vi "Dashboard Main.vi"() -> ()   [LabVIEW 2019]
uses:
  <vilib>/Rock Robotics/Network Tables/NT Read Numeric Array.vi
  <vilib>/Rock Robotics/Network Tables/NT Read String.vi
  <vilib>/Rock Robotics/Network Tables/NT Read Number.vi
  <vilib>/Rock Robotics/Network Tables/NT Read Boolean.vi
  <vilib>/Rock Robotics/Network Tables/NT Write Number.vi
panel:
  out "Camera Perf":string
  in  "Camera Settings":T1={"Frame Rate"=30, "Compression"=30, "Size"=1, "DB Camera Config"=FALSE} {"Frame Rate" scale=1.0..30.0; "Compression" scale=100.0..-1.0; "Size" items=["640x480", "320x240", "160x120"]}
  in  "TCP":refnum<k5>
  out "Robot IP":string
  in  "Dashboard Tab":T2(tab)
  in  "Select Auto":string(combo)="Select Autonomous ..."
  out "NT Connection":bool
  out "MotorChart R":cluster{"Numeric":dbl, "Numeric":dbl}(graph)
  out "MotorChart L":cluster{"Numeric":dbl, "Numeric":dbl}(graph)
  out "MotorSliders R":cluster{"MotorSlide1":dbl, "MotorSlide2":dbl} {"MotorSlide2" scale=-1.0..1.0 scale format="%#_2e"; "MotorSlide1" scale=-1.0..1.0 scale format="%#_2e"}
  out "MotorSliders L":cluster{"MotorSlide1":dbl, "MotorSlide2":dbl} {"MotorSlide2" scale=-1.0..1.0 scale format="%#_2e"; "MotorSlide1" scale=-1.0..1.0 scale format="%#_2e"}
  out "JS1 Z":dbl(slide) scale=-1.0..1.0 scale format="%#_2e"
  out "JS1 Graph":cluster{"X":dbl, "Y":dbl}[](graph)
  out "JS1 Buttons":T3
  out "JS2 Z":dbl(slide) scale=-1.0..1.0 scale format="%#_2e"
  out "JS2 Graph":cluster{"X":dbl, "Y":dbl}[](graph)
  out "JS2 Buttons":T3
  out "Mode":T4(ring)=enum."Auto Disabled"
  in  "Camera Name 2":string(combo)="No Camera Selection"
  out "Camera Image 2":T5(plugin-control)
  out "Target Spotted":bool
  out "Color Box":u32(colorbox)
  out "New Center Y":dbl
  out "New Center X":dbl
  out "y change":dbl
  out "Top Left Y":dbl
  out "Bottom Right Y":dbl
  out "Bottom Right X":dbl
  out "Top left X":dbl
  out "x change":dbl
  out "full angle":dbl
  in  "RectHeight":dbl
  in  "RectWidth":dbl
  in  "RectAngle":dbl
  in  "RectY":dbl
  in  "RectX":dbl
  out "Distance Formula 2":dbl
  out "Distance Formula 1":dbl
  out "Bottom Left Y":dbl
  out "Bottom Left X":dbl
  out "Top Right X":dbl
  out "Top Right Y":dbl
  out "New Full Angle":dbl
  out "2nd Y Change":dbl
  out "2nd X Change":dbl
  out "Final Center Y":dbl
  out "Final Center X":dbl
  out "Robot Angle":dbl
  out "Right Target":dbl
  out "Left Target":dbl
  out "Average Distance":dbl
  out "Right Distance":dbl
  out "Left Distance":dbl
  out "Right Speed":dbl
  out "Average Speed":dbl
  out "Left Speed":dbl
  out "Left":dbl[](graph)
  out "Right":dbl[](graph)
  out "Current Filter":T6 {"Value" scale=0.0..255.0; "Saturation" scale=0.0..255.0; "Hue" scale=0.0..255.0}
  in  "Update Filter":bool
  in  "New Filter":T6 {"Value" scale=0.0..255.0; "Saturation" scale=0.0..255.0; "Hue" scale=0.0..255.0}
  out "RectX":dbl
  out "RectY":dbl
  out "RectAngle":dbl
  out "RectWidth":dbl
  out "RectHeight":dbl
  out "left y":dbl
  out "right y":dbl
  out "right x":dbl
  out "left x":dbl
  in  "Update":bool
  in  "Kd":dbl format="%10.0f"
  in  "Ki":dbl format="%10.0f"
  in  "Kp":dbl format="%10.0f"
  in  "Kf":dbl format="%10.0f"
  out "Right Speed 2":dbl format="%10.0f"
  out "Left Speed 2":dbl format="%10.0f"
  out "Waveform Chart":dbl[](graph)
  in  "Right Dmd":dbl format="%10.0f"
  in  "Left Dmd":dbl format="%10.0f"
  out "Tree":string(tree)
  out "Camera Image":T5(plugin-control)
  out "Background":bool
  in  "Camera Name":string(combo)="No Camera Selection"
  # "HW"
  # "Joysticks"
  # "Drive Motors"
  # "Front"
  # "Right"
  # "Left"
  # "Back"
  # "Target Spotted"
  # "Color Sensor 90 Degree Color"
  # "Left"
  # "Right"
  # "Average"
  # "Speed"
  # "Target Speed"
  # "Distance"
  # "Robot Angle"
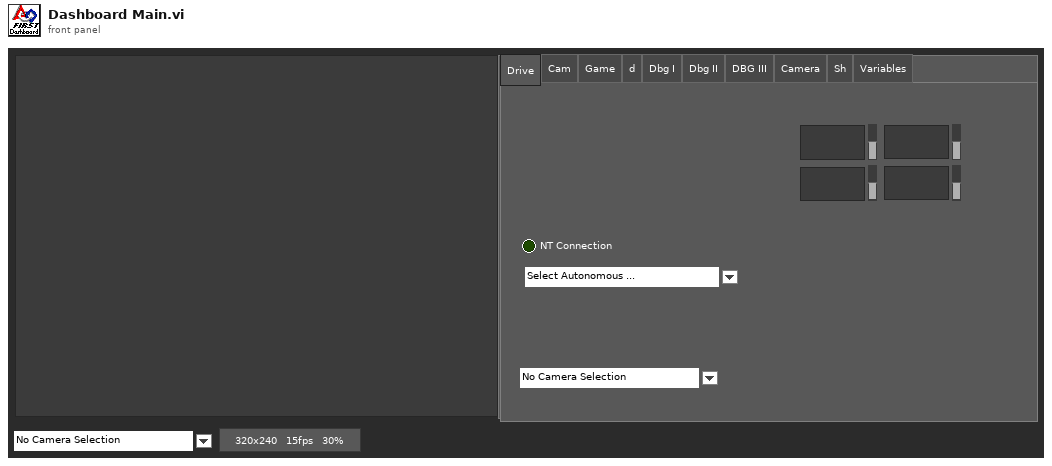
[diagram p1: front panel]
types:
  T1 = cluster{"Frame Rate":i32, "Compression":i32, "Size":u16, "DB Camera Config":bool}
  T2 = enum32{"Drive", "Cam", "Game", "d", "Dbg I", "Dbg II", "DBG III", "Camera", "Sh", "Variables"}
  T3 = cluster{bool, bool, bool, bool, bool, bool, bool, bool, bool, bool, bool, bool}
  T4 = enum8{"Tele-Op Disabled", "Tele-Op Enabled", "Auto Disabled", "Auto Enabled", "Test Disabled", "Test Enabled", "Disconnected", "No Code", "E-Stop"}
  T5 = typedef "IMAQ Image.ctl" = refnum<image>
  T6 = cluster{"Hue":cluster{dbl, dbl}, "Saturation":cluster{dbl, dbl}, "Value":cluster{dbl, dbl}}
  T7 = typedef "Image Type" = u32
  T8 = cluster{"Save Path":path, "Interval (s)":dbl, "Keep":i32}
  T9 = cluster{"Camera Image":refnum<vi>, "Dashboard Tab":refnum<vi>, "Background":refnum<vi>, "Tree":refnum<vi>, "Camera Settings":refnum<vi>, "Camera Name":refnum<vi>, "Camera Perf":refnum<vi>}
  T10 = cluster{"Shift":bool, "Ctrl":bool, "Alt":bool, "Cmd":bool, "Opt":bool}
  T11 = cluster{"Camera Name":string, "Camera File Name":string, "Saved DB Images Info":cluster{"Save Path":path, "Interval (s)":dbl, "Keep":i32}}
  T12 = cluster{"left x":dbl, "left y":dbl, "right x":dbl, "right y":dbl}
  T13 = cluster{cluster{dbl, dbl}, cluster{dbl, dbl}, cluster{dbl, dbl}}
  T14 = cluster{"left x":dbl, "right y":dbl, "right x":dbl, "left y":dbl}
  T15 = cluster{"Camera Name 2":string, string, "Saved DB Images Info":cluster{"Save Path":path, "Interval (s)":dbl, "Keep":i32}}
  T16 = cluster{"Error Strings":string, "Disable Counts":cluster{u16, u16}, "Rail Faults":cluster{u16, u16, u16}, "Robot IP":string, "DB Mode":u8, "Event Info":cluster{"Name":string, "Type":u8, "Number":u16, "Replay":u8}}
  T17 = cluster{"Storage":cluster{"Disk Free":u64, "RAM Block":u32, "RAM free":u32}, "CPU Utilization":cluster{"CPU % ISR":sgl, "CPU % Time Crit":sgl, "CPU % Timed Str":sgl, "CPU % High":sgl, "CPU % Above":sgl, "CPU % Normal":sgl, "CPU % Low":sgl}, "CAN":cluster{"% Bus Utilization":sgl, "Bus Off Cnt":u32, "TX_FIFO Full Cnt":u32, "Receive Error Cnt":u8, "Transmit Error Cnt":u8}, "HID":cluster{"HID Outputs":u32, "Rumble Low":u16, "Rumble High":u16}[]}
  T18 = cluster{"Status bits":cluster{"Test Mode":bool, "Autonomous":bool, "Enabled":bool, "Code Start":bool, "Brownout":bool, "Reserved 2":bool, "Reserved 3":bool, "E-Stop":bool}, "Code Trace":cluster{"Disabled":bool, "TeleOp":bool, "Auto":bool, "Test":bool}, "Controller Type":enum16{"unknown", "cRIO", "roboRio"}, "Code?":enum16{"unknown", "noCode", "code"}, "Battery V":dbl}
  T19 = cluster{"Control Bits":cluster{"TestMode":bool, "Autonomous":bool, "Enabled":bool, "FMS Present":bool, bool, bool, bool, "E-Stop":bool}, "Team Station ":u8, "Countdown":sgl, "Joystick Values":cluster{"Axes":dbl[], "Buttons":bool[], "POVs":i16[]}[]}
  T20 = cluster{"Axes":dbl[], "Buttons":bool[], "POVs":i16[]}[]
  T21 = cluster{"Axes":dbl[], "Buttons":bool[], "POVs":i16[]}
  T22 = cluster{"Buttons[0]":bool, "Buttons[1]":bool, "Buttons[2]":bool, "Buttons[3]":bool, "Buttons[4]":bool, "Buttons[5]":bool, "Buttons[6]":bool, "Buttons[7]":bool, "Buttons[8]":bool, "Buttons[9]":bool, "Buttons[10]":bool, "Buttons[11]":bool}
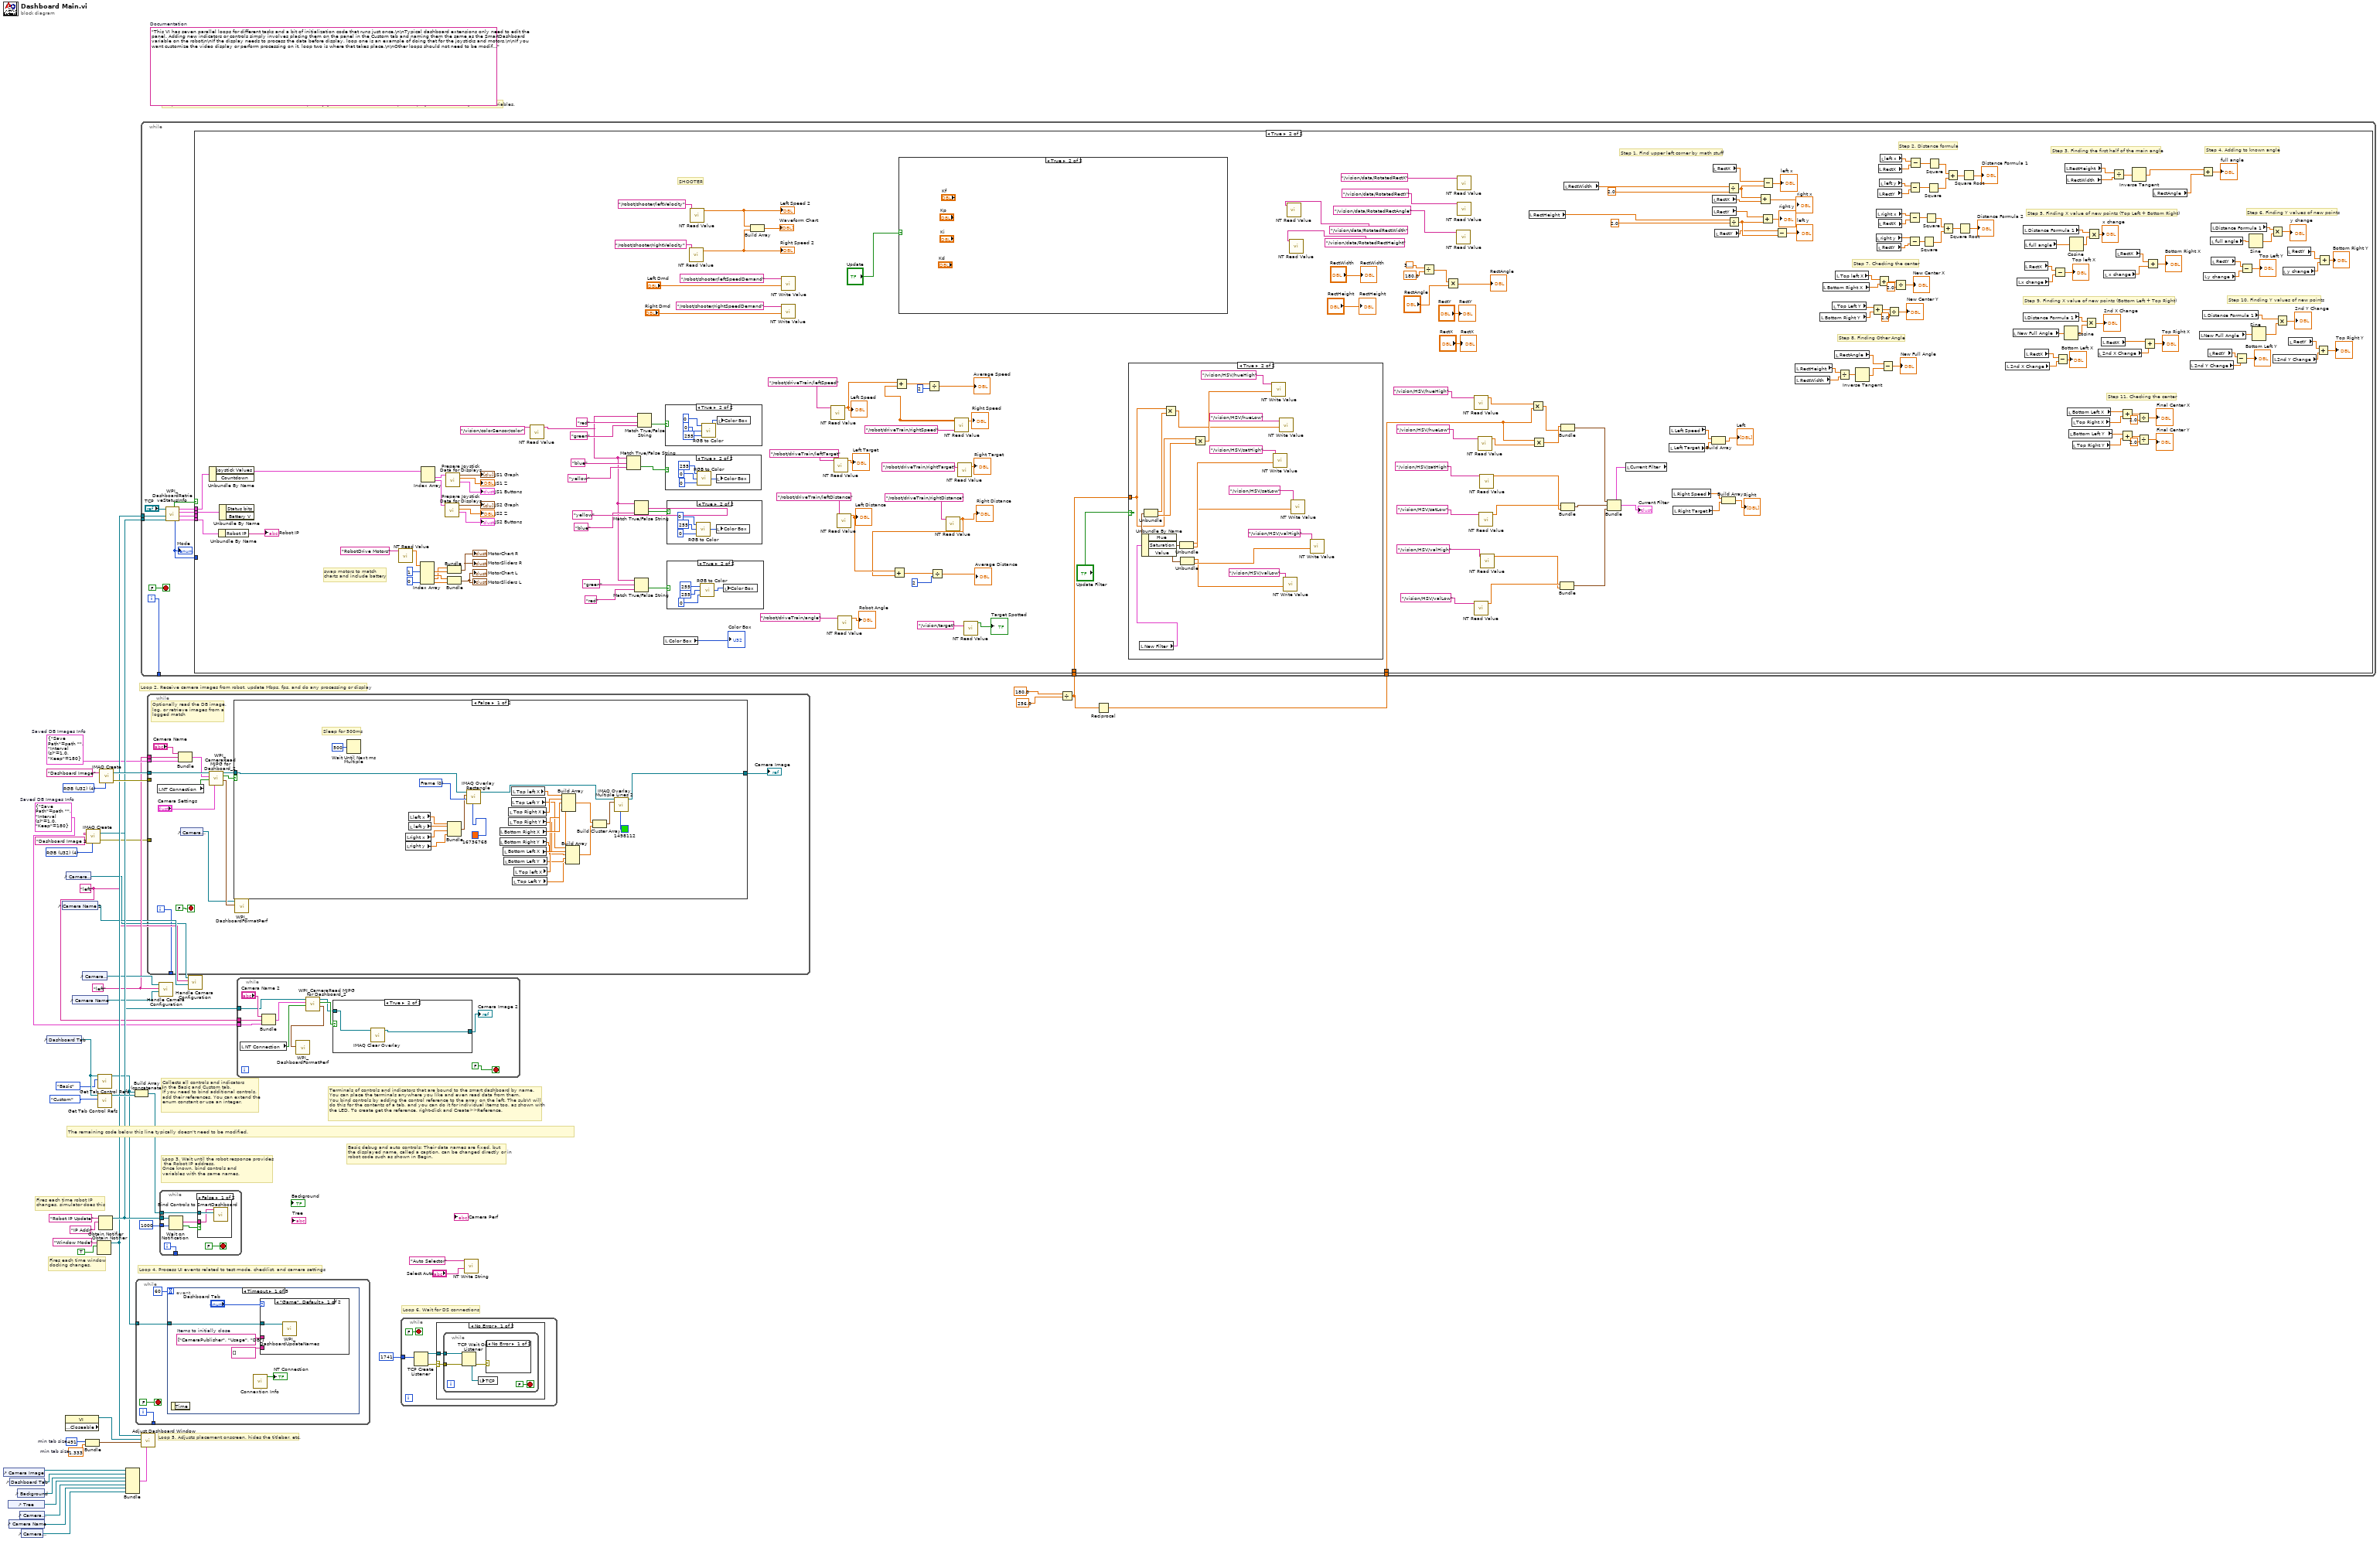
[diagram p0: block diagram]
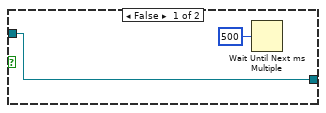
[diagram p2: hidden frame]
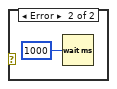
[diagram p3: hidden frame]
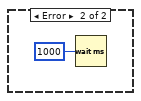
[diagram p4: hidden frame]
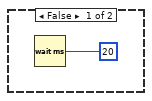
[diagram p5: hidden frame]
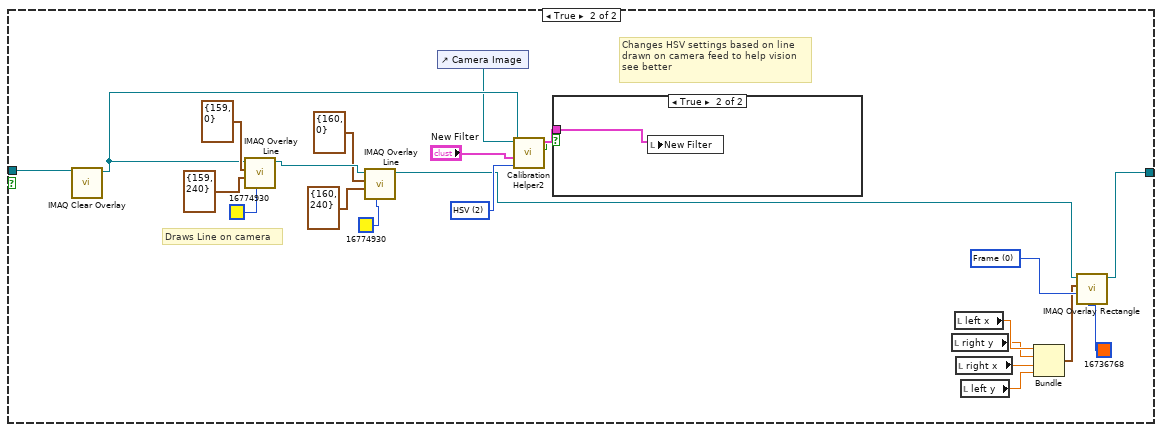
[diagram p13: hidden frame]
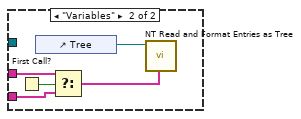
[diagram p15: hidden frame]
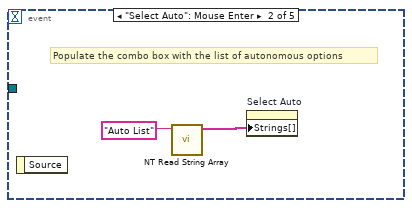
[diagram p16: hidden frame]
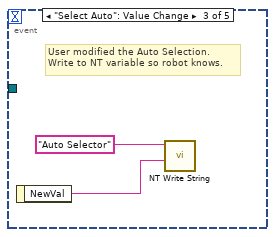
[diagram p17: hidden frame]
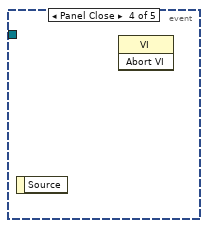
[diagram p18: hidden frame]
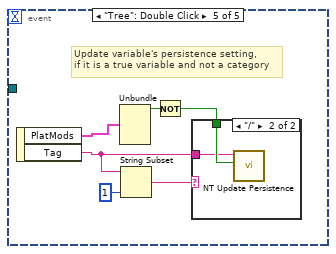
[diagram p19: hidden frame]
diagram:
  w5 = T7 4 items=["Grayscale (U8)", "Grayscale (I16)", "Grayscale (SGL)", "Complex (CSG)", "RGB (U32)", "HSL (U32)", "RGB (U64)"] ("Image Type")
  w2 = T8 {"Save Path"=path "", "Interval (s)"=1.0, "Keep"=180}  # Saved DB Images Info
  w3 = "left"
  w13 = "left" ("Camera File Name")
  w14 = T8 {"Save Path"=path "", "Interval (s)"=1.0, "Keep"=180}  # Saved DB Images Info
  w33 = 491  # min tab size
  w32 = 1.333  # min tab size
  (unwired) "This VI has seven parallel loops for different tasks and a bit of initialization code that runs just once.\n\nTypical dashboard extensions only need to edit the panel. Adding new indicators or controls simply involves placing them on the panel in the Custom tab and naming them the same as the SmartDashboard variable on the robot\n\nIf the display needs to process the data before display, loop one is an example of doing that for the joysticks and motors.\n\nIf you want customize the video display or perform processing on it, loop two is where that takes place.\n\nOther loops should not need to be modified. They are pretty standard, and document the task they perform."  # Documentation
  w48 = T7 4 items=["Grayscale (U8)", "Grayscale (I16)", "Grayscale (SGL)", "Complex (CSG)", "RGB (U32)", "HSL (U32)", "RGB (U64)"] ("Image Type")
  # "Terminals of controls and indicators that are bound to the smart dashboard by name.\nYou can place the terminals anywhere you like and even read data from them.\nYou bind controls by adding the control reference to the array on the left. The subVI will\ndo this for the contents of a tab, and you can do it for individual items too, as shown with\nthe LED. To create get the reference, right-click and Create>>Reference."
  # "Loop 6. Wait for DS connections"
  # "Basic debug and auto controls: Their data names are fixed, but\nthe displayed name, called a caption, can be changed directly or in\nrobot code such as shown in Begin."
  # "Fires each time robot IP\nchanges, simulator does this"
  # "Fires each time window\ndocking changes."
  # "Collects all controls and indicators\nin the Basic and Custom tab.\nIf you need to bind additional controls,\nadd their references. You can extend the\nenum constant or use an integer."
  # "The remaining code below this line typically doesn't need to be modified."
  # "Loop 4. Process UI events related to test mode, checklist, and camera settings"
  # "Loop 3. Wait until the robot response provides\n the Robot IP address.\nOnce known, bind controls and\nvariables with the same names."
  # "Loop 5. Adjusts placement onscreen, hides the titlebar, etc."
  # "Loop 1. Receive various data streams from Driver Station, update joystick, motors, and more complex displays that don't easily bind to variables."
  # "Loop 2. Receive camera images from robot, update Mbps, fps, and do any processing or display"
  n1 = control-ref of="Camera Image"() -> (w35:refnum<vi>)
  n2 = control-ref of="Tree"() -> (w20:refnum<vi>)
  n3 = control-ref of="Camera Name"() -> (w18:refnum<vi>)
  n4 = control-ref of="Dashboard Tab"() -> (w34:refnum<vi>)
  n5 = control-ref of="Background"() -> (w30:refnum<vi>)
  n6 = control-ref of="Camera Settings"() -> (w19:refnum<vi>)
  n7 = control-ref of="Camera Perf"() -> (w17:refnum<vi>)
  n8 = control-ref of="Dashboard Tab"() -> (w38:refnum<vi>)
  n9 = control-ref of="Camera Name 2"() -> (w8:refnum<vi>)
  n10 = property class="VI" props=["Front Panel.Closeable"]() -> (reference out=w39:refnum<vi>)  [unwired: 2 in, 2 out]
  n11 = control-ref of="Camera Settings"() -> (w7:refnum<vi>)
  n12 = control-ref of="Camera Name"() -> (w24:refnum<vi>)
  n13 = control-ref of="Camera Settings"() -> (w25:refnum<vi>)
  n14 = Bundle("min tab size"=w33, "min tab size"=w32) -> (w31:cluster{"min tab size":i32, "min tab size":dbl})  [unwired: 1 in]
  n15 = call "IMAQ Create"("Image Name"="Dashboard Image 2", "Image Type"=w5) -> ("New Image"=w1:T5, "error out"=w4:errorcluster)  [unwired: 2 in, 1 out]
  n16 = Obtain Notifier(name (unnamed)="Window Mode", notification data type=TRUE) -> (notifier out=w27:refnum<notifier>)  [unwired: 2 in, 2 out]
  n17 = call <vilib>:"Get Tab Control Refs.vi"("Page Index"=enum32{"Drive", "Basic", "Custom", "Variables"}."Basic" ("Dashboard Tab"), "TabControl in"=w38) -> ("ControlsOnPage"=w23:refnum<vi>[])  [unwired: 9 in]
  n18 = call <vilib>:"Get Tab Control Refs.vi"("Page Index"=enum32{"Drive", "Basic", "Custom", "Variables"}."Custom" ("Dashboard Tab"), "TabControl in"=w38) -> ("ControlsOnPage"=w37:refnum<vi>[])  [unwired: 9 in]
  n19 = Obtain Notifier(name (unnamed)="Robot IP Update", notification data type="IP Addr" ("name (unnamed)")) -> (notifier out=w28:refnum<notifier>)  [unwired: 2 in, 2 out]
  n20 = call "IMAQ Create"("Image Name"="Dashboard Image", "Image Type"=w48) -> ("New Image"=w46:T5, "error out"=w45:errorcluster)  [unwired: 2 in, 1 out]
  n21 = Bundle("Camera Image"=w35, "Dashboard Tab"=w34, "Background"=w30, "Tree"=w20, "Camera Settings"=w19, "Camera Name"=w18, "Camera Perf"=w17) -> (w29:T9)  [unwired: 1 in]
  n22 = Build Array (concatenate)(w23, w37) -> (w36:refnum<vi>[])
  n23 = while {
    tunnel: [w50] -> _
    tunnel: w23 -> [w49]
    i -> [w50]
    stop <- FALSE stop-if-true
    n24 = event shown="[0] Timeout" {
      selector: _ -> [_ _ _ _ _]
      dyn-events: _ -> [_ _ _ _ _]
      timeout: u32 60 ("milliseconds to wait") -> [_ _ _ _ _]
      tunnel: w49 -> [w55 _ _ _ _]
      event Timeout {
        w54 = string[] ["CameraPublisher", "Usage", "DB"]  # Items to initially close
        n25 = event-data() -> ()  [unwired: 1 in, 1 out]
        n26 = call <vilib>:"Connextion Info.vi"() -> ("Connected"=→"NT Connection":bool)  [unwired: 10 in, 1 out]
        n27 = case shown="\"Game\", Default" "Dashboard Tab" {
          tunnel: w55 -> [w58 _]
          tunnel: w54 -> [_ w61]
          tunnel: string[] [] -> [_ w60]
          frame "Game", Default {
            n28 = call <vilib>:"WPI_DashboardUpdateNames.vi"("Controls on Tab"=w58) -> ()  [unwired: 11 in]
          }
          frame "Variables" {
            n29 = First Call?() -> (First Call?: T/F=w62:bool)
            n30 = control-ref of="Tree"() -> (w63:refnum<vi>)
            n31 = Select(t=w61, s=w62, f=w60) -> (s? t:f=w59:string[])
            n32 = call <vilib>:"NT Read and Format Entries as Tree.vi"("Tags to  Close"=w59, "Tree Refnum"=w63) -> ()  [unwired: 8 in, 2 out]
          }
        }
      }
      event "Select Auto": Mouse Enter {
        # "Populate the combo box with the list of autonomous options"
        n33 = event-data() -> ()  [unwired: 1 in, 1 out]
        n34 = call <vilib>:"NT Read String Array.vi"("Name"="Auto List") -> ("String Array"=w64:string[])  [unwired: 9 in, 1 out]
        n35 = property on="Select Auto" class="CmbBox"("Strings[]"=w64) -> ()  [unwired: 2 in, 2 out]
      }
      event "Select Auto": Value Change {
        # "User modified the Auto Selection.\nWrite to NT variable so robot knows."
        n36 = event-data() -> ("NewVal"=w66:string)  [unwired: 1 in]
        n37 = call <vilib>:"NT Write String.vi"("String"=w66, "Name"="Auto Selector") -> ()  [unwired: 9 in, 1 out]
      }
      event Panel Close {
        n38 = event-data() -> ()  [unwired: 1 in, 1 out]
        n39 = invoke class="VI" method="Abort VI"() -> ()  [unwired: 3 in, 3 out]
      }
      event "Tree": Double Click {
        # "Update variable's persistence setting,\nif it is a true variable and not a category"
        n40 = event-data() -> ("PlatMods"=w69:T10, "Tag"=w68:string)  [unwired: 1 in]
        n41 = Unbundle(w69) -> ("Shift"=w73:bool)  [unwired: 4 out]
        n42 = String Subset(string=w68, length (rest)=1 ("length (rest)")) -> (substring=w70:string)  [unwired: 1 in]
        n43 = Not(x=w73) -> (.not. x?=w72:bool)
        n44 = case shown="\"/\"" w70 {
          tunnel: w72 -> [_ w75]
          tunnel: w68 -> [_ w74]
          frame Default {
          }
          frame "/" {
            n45 = call <vilib>:"NT Update Persistence.vi"("Persistence"=w75, "Name"=w74) -> ()  [unwired: 9 in, 1 out]
          }
        }
      }
    }
  }
  n46 = call "Adjust Dashboard Window.vi"("Sizing Refnums"=w29, "Size Constraints"=w31, "VI"=w39, "WIn Mode"=w27) -> ()  [unwired: 8 in]
  n47 = while {
    tunnel: w46 -> [w87]
    tunnel: w45 -> [_]
    tunnel: [w88] -> _
    tunnel: w14 -> [w82]
    tunnel: w13 -> [w79]
    tunnel: w4 -> [_]
    i -> [w88]
    stop <- FALSE stop-if-true
    # "Optionally read the DB image,\nlog, or retrieve images from a\nlogged match"
    n48 = local read "NT Connection"() -> (w83:bool)
    n49 = Bundle("Camera Name"="Camera Name", "Camera File Name"=w79, "Saved DB Images Info"=w82) -> (w81:T11)  [unwired: 1 in]
    n50 = control-ref of="Camera Perf"() -> (w77:refnum<vi>)
    n51 = call <vilib>:"WPI_CameraRead MJPG for Dashboard_2.vi"("Camera Settings"="Camera Settings", "NT Connection"=w83, "Capture Info"=w81, "Image in"=w87) -> ("perf info"=w78:cluster{"Bandwidth (Mbps)":dbl, "fps":dbl}, "Active"=w86:bool, "Image\\ out"=w76:T5)  [unwired: 5 in]
    n52 = case shown="False" w86 {
      tunnel: [w91 w117] -> w84
      tunnel: w76 -> [w112 w134]
      frame False {
        w113 = u32 0 items=["Frame", "Fill", "Highlight"] ("Drawing Mode (Frame)")
        # "Sleep for 500ms"
        n53 = Wait Until Next ms Multiple(millisecond multiple=u32 500) -> ()  [unwired: 1 out]
        n54 = local read "right x"() -> (w107:dbl)
        n55 = local read "right y"() -> (w106:dbl)
        n56 = local read "left x"() -> (w109:dbl)
        n57 = local read "left y"() -> (w108:dbl)
        n58 = Bundle("left x"=w109, "left y"=w108, "right x"=w107, "right y"=w106) -> (w110:T12)  [unwired: 1 in]
        n59 = call "IMAQ Overlay Rectangle"("Color"=u32 16736768, "Drawing Mode (Frame)"=w113, "Rectangle"=w110, "Image"=w112) -> ("Image Out"=w92:T5)  [unwired: 6 in, 1 out]
        n60 = local read "Bottom Right X"() -> (w103:dbl)
        n61 = local read "Bottom Right Y"() -> (w98:dbl)
        n62 = local read "Bottom Left X"() -> (w102:dbl)
        n63 = local read "Bottom Left Y"() -> (w97:dbl)
        n64 = local read "Top Right X"() -> (w104:dbl)
        n65 = local read "Top Right Y"() -> (w99:dbl)
        n66 = local read "Top Left Y"() -> (w100:dbl)
        n67 = local read "Top left X"() -> (w105:dbl)
        n68 = local read "Top Left Y"() -> (w96:dbl)
        n69 = local read "Top left X"() -> (w101:dbl)
        n70 = Build Array(w105, w104, w103, w102, w101) -> (w95:dbl[])
        n71 = Build Array(w100, w99, w98, w97, w96) -> (w94:dbl[])
        n72 = Build Cluster Array(w95, w94) -> (w93:cluster{"Top left X":dbl, "Top Left Y":dbl}[])
        n73 = call "IMAQ Overlay Multiple Lines 2"("Image"=w92, "Line End Points"=w93, "Color"=u32 1498112) -> ("Image Out"=w91:T5)  [unwired: 11 in, 1 out]
      }
      frame True {
        w124 = u32 0 items=["Frame", "Fill", "Highlight"] ("Drawing Mode (Frame)")
        w132 = u16 2 items=["RGB", "HSL", "HSV", "HSI", "CIE L*a*b*", "CIE XYZ"] ("Color Mode")
        # "Changes HSV settings based on line drawn on camera feed to help vision see better"
        # "Draws Line on camera"
        n74 = call "IMAQ Clear Overlay"("Image"=w134) -> ("Image Out"=w133:T5)  [unwired: 2 in, 8 out]
        n75 = call "IMAQ Overlay Line"("Color"=u32 16774930, "End Point"=cluster{i32, i32} {159, 240}, "Start Point"=cluster{i32, i32} {159, 0}, "Image"=w133) -> ("Image Out"=w128:T5)  [unwired: 6 in, 1 out]
        n76 = call "IMAQ Overlay Line"("Color"=u32 16774930, "End Point"=cluster{i32, i32} {160, 240}, "Start Point"=cluster{i32, i32} {160, 0}, "Image"=w128) -> ("Image Out"=w118:T5)  [unwired: 6 in, 1 out]
        n77 = control-ref of="Camera Image"() -> (w115:refnum<vi>)
        n78 = call "Calibration Helper2.vi"("Color Mode"=w132, "Color Components"="New Filter", "Image"=w133, "Image Ctl Refnum"=w115) -> ("Changed"=w130:bool, "output color"=w131:T13)  [unwired: 6 in]
        n79 = case shown="True" w130 {
          tunnel: w131 -> [_ w138]
          frame False {
          }
          frame True {
            n80 = local write "New Filter"(w138) -> ()
          }
        }
        n81 = local read "right y"() -> (w122:dbl)
        n82 = local read "left x"() -> (w123:dbl)
        n83 = local read "right x"() -> (w121:dbl)
        n84 = local read "left y"() -> (w120:dbl)
        n85 = Bundle("left x"=w123, "right y"=w122, "right x"=w121, "left y"=w120) -> (w119:T14)  [unwired: 1 in]
        n86 = call "IMAQ Overlay Rectangle"("Color"=u32 16736768, "Drawing Mode (Frame)"=w124, "Rectangle"=w119, "Image"=w118) -> ("Image Out"=w117:T5)  [unwired: 6 in, 1 out]
      }
    }
    "Camera Image" <- w84
    n87 = call <vilib>:"WPI_DashboardFormatPerf.vi"("Performance"=w78, "String in"=w77) -> ()  [unwired: 10 in]
  }
  n88 = call "Handle Camera Configuration.vi"("CameraNameRef"=w24, "Display Name"=w13, "ClusterRef"=w25) -> ()  [unwired: 9 in]
  n89 = while {
    tunnel: w36 -> [w145]
    tunnel: w28 -> [w143]
    tunnel: [w141] -> _
    tunnel: u32 1000 ("milliseconds to wait") -> [w140]
    i -> [w141]
    stop <- FALSE stop-if-true
    n90 = Wait on Notification(notifier=w143, timeout in ms (-1)=w140) -> (notification=w142:string, timed out?=w139:bool)  [unwired: 2 in, 2 out]
    n91 = case shown="False" w139 {
      tunnel: w145 -> [w147 _]
      tunnel: w142 -> [w146 _]
      frame False {
        n92 = call <vilib>:"Bind Controls to SmartDashboard.vi"("Bound Control Refs"=w147, "Server IP Address"=w146) -> ()  [unwired: 10 in]
      }
      frame True {
      }
    }
  }
  n93 = call "Handle Camera Configuration.vi"("CameraNameRef"=w8, "Display Name"=w3, "ClusterRef"=w7) -> ()  [unwired: 9 in]
  n94 = while {
    tunnel: w3 -> [w157]
    tunnel: w2 -> [w156]
    tunnel: w1 -> [w153]
    stop <- FALSE stop-if-true
    n95 = local read "NT Connection"() -> (w148:bool)
    n96 = Bundle("Camera Name 2"="Camera Name 2", w157, "Saved DB Images Info"=w156) -> (w154:T15)  [unwired: 1 in]
    n97 = call <vilib>:"WPI_CameraRead MJPG for Dashboard_2.vi"("NT Connection"=w148, "Capture Info"=w154, "Image in"=w153) -> ("perf info"=w149:cluster{"Bandwidth (Mbps)":dbl, "fps":dbl}, "Active"=w152:bool, "Image\\ out"=w151:T5)  [unwired: 6 in]
    n98 = call <vilib>:"WPI_DashboardFormatPerf.vi"("Performance"=w149) -> ()  [unwired: 11 in]
    n99 = case shown="True" w152 {
      tunnel: w151 -> [w159 w162]
      tunnel: [w159 w161] -> w150
      frame False {
        n100 = Wait Until Next ms Multiple(millisecond multiple=u32 500) -> ()  [unwired: 1 out]
      }
      frame True {
        n101 = call "IMAQ Clear Overlay"("Image"=w162) -> ("Image Out"=w161:T5)  [unwired: 2 in, 8 out]
      }
    }
    "Camera Image 2" <- w150
  }
  n102 = while {
    tunnel: u16 1741 ("timeout ms (25000)") -> [w164]
    stop <- FALSE stop-if-true
    n103 = TCP Create Listener(10:w164) -> (0:w163:errorcluster, 3:w165:refnum<k5>)  [unwired: 4 in, 1 out]
    n104 = case shown="No Error" w163 {
      selector: w163 -> [w167 _]
      tunnel: w165 -> [w168 _]
      frame No Error {
        n105 = while {
          tunnel: w168 -> [w171]
          tunnel: w167 -> [w170]
          stop <- FALSE stop-if-true
          n106 = TCP Wait On Listener(8:w170, 11:w171) -> (0:w172:errorcluster, 4:w173:refnum<k5>)  [unwired: 2 in, 3 out]
          n107 = local write "TCP"(w173) -> ()
          n108 = case shown="No Error" w172 {
            frame No Error {
            }
            frame Error {
              n109 = Wait (ms)(milliseconds to wait=u32 1000) -> ()  [unwired: 1 out]
            }
          }
        }
      }
      frame Error {
        n110 = Wait (ms)(milliseconds to wait=u32 1000) -> ()  [unwired: 1 out]
      }
    }
  }
  n111 = call <vilib>:"NT Write String.vi"("String"="Select Auto", "Name"="Auto Selector") -> ()  [unwired: 9 in, 1 out]
  n112 = Divide(x=180.0, y=256.0) -> (x/y=w10:dbl)
  n113 = Reciprocal(x=w10) -> (1/x=w9:dbl)
  n114 = while {
    tunnel: [w187] -> _
    tunnel: w28 -> [w181]
    tunnel: w27 -> [w178]
    tunnel: w10 -> [w177]
    tunnel: w9 -> [w176]
    i -> [w187]
    stop <- FALSE stop-if-true
    n115 = call <vilib>:"WPI_DashboardRetrieveStatusInfo.vi"("Binding Refnum"=w181, "Window Mode Notifier"=w178, "TCP Cnx"="TCP") -> ("Power and Errors"=w182:T16, "Robot Metrics"=w185:T17, "Status Info"=w186:T18, "Control Info"=w183:T19, "Robot Mode"=w180:T4, "Process?"=w184:bool)  [unwired: 3 in]
    "Mode" <- w180
    n116 = case shown="True" w184 {
      tunnel: w186 -> [_ w407]
      tunnel: w185 -> [_ _]
      tunnel: w183 -> [_ w406]
      tunnel: w182 -> [_ w405]
      tunnel: w180 -> [_ _]
      tunnel: w177 -> [_ w346]
      tunnel: w176 -> [_ w337]
      frame False {
        n117 = Wait (ms)(milliseconds to wait=u32 20) -> ()  [unwired: 1 out]
      }
      frame True {
        # "Step 11. Checking the center"
        # "Step 10. Finding Y values of new points"
        # "Step 9. Finding X value of new points (Bottom Left + Top Right)"
        # "Step 8. Finding Other Angle"
        # "Step 7. Checking the center"
        # "Step 6. Finding Y values of new points"
        # "Step 5. Finding X value of new points (Top Left + Bottom Right)"
        # "Step 4. Adding to known angle"
        # "Step 3. Finding the first half of the main angle"
        # "Step 2. Distance formula"
        # "Step 1. Find upper left corner by math stuff"
        # "SHOOTER"
        # "swap motors to match\ncharts and include battery"
        n118 = Unbundle By Name(w406) -> ("Joystick Values"=w396:T20)  [unwired: 1 out]
        n119 = Unbundle By Name(w405) -> ("Robot IP"=→"Robot IP":string)
        n120 = Unbundle By Name(w407) -> ()  [unwired: 2 out]
        n121 = call-poly <vilib>:"NT Read Value.vi"("Name"="RobotDrive Motors") -> ("Numeric Array"=w386:dbl[])  [unwired: 9 in, 1 out]
        n122 = Index Array(array=w386, index #1=1, index #4=0) -> (element #1=w400:dbl, element #2=w401:dbl, element #3=w399:dbl, element #4=w404:dbl)  [unwired: 2 in]
        n123 = Index Array(array=w396) -> (element #1=w395:T21, element #2=w391:T21)  [unwired: 2 in]
        n124 = call "Prepare Joystick Data for Displays.vi"("Joystick Values"=w391) -> ("Buttons"=→"JS2 Buttons":T22, "Z Axis"=→"JS2 Z":dbl, "Cartesian Data"=→"JS2 Graph":cluster{"X axis":dbl, "X axis":dbl}[])  [unwired: 8 in]
        n125 = call "Prepare Joystick Data for Displays.vi"("Joystick Values"=w395) -> ("Buttons"=→"JS1 Buttons":T22, "Z Axis"=→"JS1 Z":dbl, "Cartesian Data"=→"JS1 Graph":cluster{"X axis":dbl, "X axis":dbl}[])  [unwired: 8 in]
        n126 = Bundle("Numeric"=w399, "Numeric"=w400) -> (→"MotorChart R" →"MotorSliders R":cluster{"Numeric":dbl, "Numeric":dbl})  [unwired: 1 in]
        n127 = Bundle("Numeric"=w401, "Numeric"=w404) -> (→"MotorChart L" →"MotorSliders L":cluster{"Numeric":dbl, "Numeric":dbl})  [unwired: 1 in]
        n128 = call-poly <vilib>:"NT Read Value.vi"("Name"="/vision/colorSensor/color") -> ("String"=w347:string)  [unwired: 9 in, 1 out]
        n129 = Match True/False String(2:"yellow" ("false string"), 3:"blue" ("true string"), 4:w347) -> (0:w373:bool)  [unwired: 1 out]
        n130 = Match True/False String(2:"blue" ("false string"), 3:"yellow" ("true string"), 4:w347) -> (0:w372:bool)  [unwired: 1 out]
        n131 = Match True/False String(2:"red" ("false string"), 3:"green" ("true string"), 4:w347) -> (0:w382:bool)  [unwired: 1 out]
        n132 = Match True/False String(2:"green" ("false string"), 3:"red" ("true string"), 4:w347) -> (0:w383:bool)  [unwired: 1 out]
        n133 = local read "Color Box"() -> (→"Color Box":u32)
        n134 = case shown="True" w383 {
          frame False {
          }
          frame True {
            n135 = call <vilib>:"RGB to Color.vi"("B"=255, "G"=0, "R"=0) -> ("Color"=w439:u32)
            n136 = local write "Color Box"(w439) -> ()
          }
        }
        n137 = case shown="True" w373 {
          frame False {
          }
          frame True {
            n138 = call <vilib>:"RGB to Color.vi"("B"=0, "G"=0, "R"=255) -> ("Color"=w431:u32)
            n139 = local write "Color Box"(w431) -> ()
          }
        }
        n140 = case shown="True" w372 {
          frame False {
          }
          frame True {
            n141 = call <vilib>:"RGB to Color.vi"("B"=0, "G"=255, "R"=0) -> ("Color"=w427:u32)
            n142 = local write "Color Box"(w427) -> ()
          }
        }
        n143 = case shown="True" w382 {
          frame False {
          }
          frame True {
            n144 = call <vilib>:"RGB to Color.vi"("B"=0, "G"=255, "R"=255) -> ("Color"=w435:u32)
            n145 = local write "Color Box"(w435) -> ()
          }
        }
        n146 = call-poly <vilib>:"NT Read Value.vi"("Name"="/robot/shooter/rightVelocity") -> ("Numeric"=w317:dbl)  [unwired: 9 in, 1 out]
        "Right Speed 2" <- w317
        n147 = call-poly <vilib>:"NT Read Value.vi"("Name"="/robot/shooter/leftVelocity") -> ("Numeric"=w318:dbl)  [unwired: 9 in, 1 out]
        "Left Speed 2" <- w318
        n148 = Build Array(w318, w317) -> (→"Waveform Chart":dbl[])
        n149 = call-poly <vilib>:"NT Write Value.vi"("Numeric"="Right Dmd", "Name"="/robot/shooter/rightSpeedDemand") -> ()  [unwired: 9 in, 1 out]
        n150 = call-poly <vilib>:"NT Write Value.vi"("Numeric"="Left Dmd", "Name"="/robot/shooter/leftSpeedDemand") -> ()  [unwired: 9 in, 1 out]
        n151 = call-poly <vilib>:"NT Read Value.vi"("Name"="/robot/driveTrain/leftSpeed") -> ("Numeric"=w362:dbl)  [unwired: 9 in, 1 out]
        "Left Speed" <- w362
        n152 = call-poly <vilib>:"NT Read Value.vi"("Name"="/robot/driveTrain/leftTarget") -> ("Numeric"=→"Left Target":dbl)  [unwired: 9 in, 1 out]
        n153 = call-poly <vilib>:"NT Read Value.vi"("Name"="/robot/driveTrain/leftDistance") -> ("Numeric"=w357:dbl)  [unwired: 9 in, 1 out]
        "Left Distance" <- w357
        n154 = call-poly <vilib>:"NT Read Value.vi"("Name"="/robot/driveTrain/angle") -> ("Numeric"=→"Robot Angle":dbl)  [unwired: 9 in, 1 out]
        n155 = case shown="True" "Update" {
          frame False {
          }
          frame True {
          }
        }
        n156 = call-poly <vilib>:"NT Read Value.vi"("Name"="/robot/driveTrain/rightDistance") -> ("Numeric"=w356:dbl)  [unwired: 9 in, 1 out]
        "Right Distance" <- w356
        n157 = Add(x=w357, y=w356) -> (x+y=w355:dbl)
        n158 = Divide(x=w355, y=2) -> (x/y=→"Average Distance":dbl)
        n159 = call-poly <vilib>:"NT Read Value.vi"("Name"="/robot/driveTrain/rightSpeed") -> ("Numeric"=w361:dbl)  [unwired: 9 in, 1 out]
        "Right Speed" <- w361
        n160 = Add(x=w362, y=w361) -> (x+y=w360:dbl)
        n161 = Divide(x=w360, y=2) -> (x/y=→"Average Speed":dbl)
        n162 = call-poly <vilib>:"NT Read Value.vi"("Name"="/robot/driveTrain/rightTarget") -> ("Numeric"=→"Right Target":dbl)  [unwired: 9 in, 1 out]
        n163 = call-poly <vilib>:"NT Read Value.vi"("Name"="/vision/target") -> ("Boolean"=→"Target Spotted":bool)  [unwired: 9 in, 1 out]
        n164 = case shown="True" "Update Filter" {
          tunnel: w346 -> [_ w415]
          frame False {
          }
          frame True {
            n165 = local read "New Filter"() -> (w414:T6)
            n166 = Unbundle By Name(w414) -> ("Hue"=w426:cluster{dbl, dbl}, "Saturation"=w425:cluster{dbl, dbl}, "Value"=w424:cluster{dbl, dbl})
            n167 = Unbundle(w426) -> (w417:dbl, w416:dbl)
            n168 = Multiply(x=w415, y=w417) -> (x*y=w412:dbl)
            n169 = Unbundle(w425) -> (w410:dbl, w411:dbl)
            n170 = Unbundle(w424) -> (w408:dbl, w409:dbl)
            n171 = Multiply(x=w415, y=w416) -> (x*y=w413:dbl)
            n172 = call-poly <vilib>:"NT Write Value.vi"("Numeric"=w413, "Name"="/vision/HSV/hueHigh") -> ()  [unwired: 9 in, 1 out]
            n173 = call-poly <vilib>:"NT Write Value.vi"("Numeric"=w411, "Name"="/vision/HSV/satHigh") -> ()  [unwired: 9 in, 1 out]
            n174 = call-poly <vilib>:"NT Write Value.vi"("Numeric"=w412, "Name"="/vision/HSV/hueLow") -> ()  [unwired: 9 in, 1 out]
            n175 = call-poly <vilib>:"NT Write Value.vi"("Numeric"=w408, "Name"="/vision/HSV/valLow") -> ()  [unwired: 9 in, 1 out]
            n176 = call-poly <vilib>:"NT Write Value.vi"("Numeric"=w410, "Name"="/vision/HSV/satLow") -> ()  [unwired: 9 in, 1 out]
            n177 = call-poly <vilib>:"NT Write Value.vi"("Numeric"=w409, "Name"="/vision/HSV/valHigh") -> ()  [unwired: 9 in, 1 out]
          }
        }
        n178 = call-poly <vilib>:"NT Read Value.vi"("Name"="/vision/data/RotatedRectWidth") -> ()  [unwired: 9 in, 2 out]
        n179 = call-poly <vilib>:"NT Read Value.vi"("Name"="/vision/data/RotatedRectHeight") -> ()  [unwired: 9 in, 2 out]
        n180 = Divide(x=3.141592653589793, y=180.0) -> (x/y=w259:dbl)
        n181 = Multiply(x=w259, y="RectAngle") -> (x*y=→"RectAngle":dbl)
        n182 = call-poly <vilib>:"NT Read Value.vi"("Name"="/vision/data/RotatedRectAngle") -> ()  [unwired: 9 in, 2 out]
        n183 = call-poly <vilib>:"NT Read Value.vi"("Name"="/vision/data/RotatedRectX") -> ()  [unwired: 9 in, 2 out]
        n184 = call-poly <vilib>:"NT Read Value.vi"("Name"="/vision/data/RotatedRectY") -> ()  [unwired: 9 in, 2 out]
        n185 = call-poly <vilib>:"NT Read Value.vi"("Name"="/vision/HSV/hueHigh") -> ("Numeric"=w339:dbl)  [unwired: 9 in, 1 out]
        n186 = call-poly <vilib>:"NT Read Value.vi"("Name"="/vision/HSV/valLow") -> ("Numeric"=w327:dbl)  [unwired: 9 in, 1 out]
        n187 = call-poly <vilib>:"NT Read Value.vi"("Name"="/vision/HSV/hueLow") -> ("Numeric"=w338:dbl)  [unwired: 9 in, 1 out]
        n188 = call-poly <vilib>:"NT Read Value.vi"("Name"="/vision/HSV/satLow") -> ("Numeric"=w328:dbl)  [unwired: 9 in, 1 out]
        n189 = call-poly <vilib>:"NT Read Value.vi"("Name"="/vision/HSV/satHigh") -> ("Numeric"=w329:dbl)  [unwired: 9 in, 1 out]
        n190 = call-poly <vilib>:"NT Read Value.vi"("Name"="/vision/HSV/valHigh") -> ("Numeric"=w326:dbl)  [unwired: 9 in, 1 out]
        n191 = local read "RectHeight"() -> (w293:dbl)
        n192 = Multiply(x=w339, y=w337) -> (x*y=w330:dbl)
        n193 = Multiply(x=w337, y=w338) -> (x*y=w331:dbl)
        n194 = Bundle("Numeric"=w327, "Numeric"=w326) -> (w332:cluster{"Numeric":dbl, "Numeric":dbl})  [unwired: 1 in]
        n195 = Bundle(w331, w330) -> (w334:cluster{dbl, dbl})  [unwired: 1 in]
        n196 = Bundle("Numeric"=w328, "Numeric"=w329) -> (w333:cluster{"Numeric":dbl, "Numeric":dbl})  [unwired: 1 in]
        n197 = local read "RectWidth"() -> (w294:dbl)
        n198 = local read "Current Filter"() -> (w335:T6)
        n199 = Bundle(cluster=w335, "Hue"=w334, "Saturation"=w333, "Value"=w332) -> (→"Current Filter":T6)
        n200 = local read "Left Target"() -> (w309:dbl)
        n201 = local read "Left Speed"() -> (w310:dbl)
        n202 = local read "Right Speed"() -> (w306:dbl)
        n203 = local read "Right Target"() -> (w307:dbl)
        n204 = Build Array(w310, w309) -> (→"Left":dbl[])
        n205 = local read "RectX"() -> (w300:dbl)
        n206 = local read "RectY"() -> (w297:dbl)
        n207 = local read "RectX"() -> (w295:dbl)
        n208 = local read "RectY"() -> (w296:dbl)
        n209 = Build Array(w306, w307) -> (→"Right":dbl[])
        n210 = Divide(x=w294, y=2.0) -> (x/y=w299:dbl)
        n211 = Divide(x=w293, y=2.0) -> (x/y=w298:dbl)
        n212 = Add(x=w299, y=w300) -> (x+y=→"right x":dbl)
        n213 = Add(x=w297, y=w298) -> (x+y=→"right y":dbl)
        n214 = Subtract(x=w295, y=w299) -> (x-y=→"left x":dbl)
        n215 = Subtract(x=w296, y=w298) -> (x-y=→"left y":dbl)
        n216 = local read "RectHeight"() -> (w223:dbl)
        n217 = local read "RectWidth"() -> (w225:dbl)
        n218 = local read "Bottom Right Y"() -> (w230:dbl)
        n219 = local read "Bottom Right X"() -> (w234:dbl)
        n220 = local read "Top Left Y"() -> (w231:dbl)
        n221 = local read "RectAngle"() -> (w222:dbl)
        n222 = local read "Top left X"() -> (w235:dbl)
        n223 = Divide(x=w223, y=w225) -> (x/y=w224:dbl)
        n224 = Inverse Tangent(1:w224) -> (0:w221:dbl)
        n225 = Add(x=w231, y=w230) -> (x+y=w229:dbl)
        n226 = local read "right y"() -> (w278:dbl)
        n227 = local read "right x"() -> (w280:dbl)
        n228 = local read "RectY"() -> (w277:dbl)
        n229 = Add(x=w235, y=w234) -> (x+y=w233:dbl)
        n230 = local read "RectY"() -> (w281:dbl)
        n231 = local read "RectX"() -> (w289:dbl)
        n232 = local read "RectX"() -> (w279:dbl)
        n233 = local read "left y"() -> (w288:dbl)
        n234 = local read "left x"() -> (w290:dbl)
        n235 = Subtract(x=w222, y=w221) -> (x-y=→"New Full Angle":dbl)
        n236 = Divide(x=w229, y=2.0) -> (x/y=→"New Center Y":dbl)
        n237 = Divide(x=w233, y=2.0) -> (x/y=→"New Center X":dbl)
        n238 = Subtract(x=w280, y=w279) -> (x-y=w276:dbl)
        n239 = Subtract(x=w278, y=w277) -> (x-y=w275:dbl)
        n240 = Subtract(x=w288, y=w281) -> (x-y=w286:dbl)
        n241 = Subtract(x=w290, y=w289) -> (x-y=w287:dbl)
        n242 = Square(x=w275) -> (x^2=w273:dbl)
        n243 = Square(x=w276) -> (x^2=w274:dbl)
        n244 = Square(x=w286) -> (x^2=w284:dbl)
        n245 = Square(x=w287) -> (x^2=w285:dbl)
        n246 = Add(x=w274, y=w273) -> (x+y=w272:dbl)
        n247 = Add(x=w285, y=w284) -> (x+y=w283:dbl)
        n248 = Square Root(x=w272) -> (sqrt(x)=→"Distance Formula 2":dbl)
        n249 = Square Root(x=w283) -> (sqrt(x)=→"Distance Formula 1":dbl)
        n250 = local read "2nd X Change"() -> (w214:dbl)
        n251 = local read "New Full Angle"() -> (w219:dbl)
        n252 = local read "x change"() -> (w250:dbl)
        n253 = local read "Distance Formula 1"() -> (w217:dbl)
        n254 = local read "Distance Formula 1"() -> (w255:dbl)
        n255 = local read "full angle"() -> (w254:dbl)
        n256 = local read "RectX"() -> (w251:dbl)
        n257 = local read "RectX"() -> (w215:dbl)
        n258 = Subtract(x=w251, y=w250) -> (x-y=→"Top left X":dbl)
        n259 = Subtract(x=w215, y=w214) -> (x-y=→"Bottom Left X":dbl)
        n260 = Cosine(x=w219) -> (cos(x)=w218:dbl)
        n261 = local read "RectHeight"() -> (w266:dbl)
        n262 = local read "RectWidth"() -> (w265:dbl)
        n263 = local read "Bottom Left X"() -> (w195:dbl)
        n264 = local read "Bottom Left Y"() -> (w192:dbl)
        n265 = Cosine(x=w254) -> (cos(x)=w253:dbl)
        n266 = local read "Top Right X"() -> (w193:dbl)
        n267 = local read "Top Right Y"() -> (w191:dbl)
        n268 = Multiply(x=w217, y=w218) -> (x*y=→"2nd X Change":dbl)
        n269 = Multiply(x=w255, y=w253) -> (x*y=→"x change":dbl)
        n270 = local read "2nd X Change"() -> (w212:dbl)
        n271 = local read "RectX"() -> (w211:dbl)
        n272 = local read "x change"() -> (w247:dbl)
        n273 = Divide(x=w266, y=w265) -> (x/y=w264:dbl)
        n274 = local read "RectX"() -> (w248:dbl)
        n275 = Add(x=w195, y=w193) -> (x+y=w199:dbl)
        n276 = Add(x=w192, y=w191) -> (x+y=w197:dbl)
        n277 = Inverse Tangent(1:w264) -> (0:w258:dbl)
        n278 = Divide(x=w199, y=2.0) -> (x/y=→"Final Center X":dbl)
        n279 = Divide(x=w197, y=2.0) -> (x/y=→"Final Center Y":dbl)
        n280 = Add(x=w211, y=w212) -> (x+y=→"Top Right X":dbl)
        n281 = Add(x=w248, y=w247) -> (x+y=→"Bottom Right X":dbl)
        n282 = local read "RectAngle"() -> (w257:dbl)
        n283 = local read "2nd Y Change"() -> (w204:dbl)
        n284 = local read "New Full Angle"() -> (w209:dbl)
        n285 = Add(x=w258, y=w257) -> (x+y=→"full angle":dbl)
        n286 = local read "Distance Formula 1"() -> (w207:dbl)
        n287 = local read "y change"() -> (w240:dbl)
        n288 = local read "RectY"() -> (w205:dbl)
        n289 = local read "full angle"() -> (w243:dbl)
        n290 = local read "Distance Formula 1"() -> (w245:dbl)
        n291 = local read "RectY"() -> (w241:dbl)
        n292 = Subtract(x=w205, y=w204) -> (x-y=→"Bottom Left Y":dbl)
        n293 = Subtract(x=w241, y=w240) -> (x-y=→"Top Left Y":dbl)
        n294 = Sine(x=w243) -> (sin(x)=w244:dbl)
        n295 = Sine(x=w209) -> (sin(x)=w208:dbl)
        n296 = Multiply(x=w245, y=w244) -> (x*y=→"y change":dbl)
        n297 = local read "2nd Y Change"() -> (w201:dbl)
        n298 = Multiply(x=w207, y=w208) -> (x*y=→"2nd Y Change":dbl)
        n299 = local read "y change"() -> (w237:dbl)
        n300 = local read "RectY"() -> (w238:dbl)
        n301 = local read "RectY"() -> (w202:dbl)
        n302 = Add(x=w202, y=w201) -> (x+y=→"Top Right Y":dbl)
        n303 = Add(x=w238, y=w237) -> (x+y=→"Bottom Right Y":dbl)
        "RectX" <- "RectX"
        "RectY" <- "RectY"
        "RectWidth" <- "RectWidth"
        "RectHeight" <- "RectHeight"
      }
    }
  }
